vi "Create Response Description.vi"(8 "error in (no error)":errorcluster, 10 "JSON in":string, 11 "Help in":refnum<class "Help.lvclass">) -> (0 "error out":errorcluster, 2 "<JSON> out":string, 3 "Help out":refnum<class "Help.lvclass">)   [LabVIEW 2019, in "Instrument.lvlib" / "Help.lvclass"]
uses:
  Help.lvclass
  Help.lvclass/Help.ctl
  <vilib>/ciozi137/JSON-Schema/API/Read Typedef Description (variant).vi
  <vilib>/JDP Science/JSONtext/JSONtext.lvlib
  <vilib>/ciozi137/JSON-Schema/JSON-Schema.lvlib
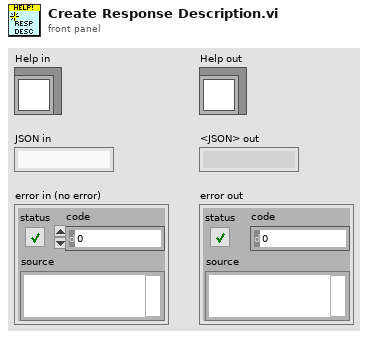
[diagram p1: front panel]
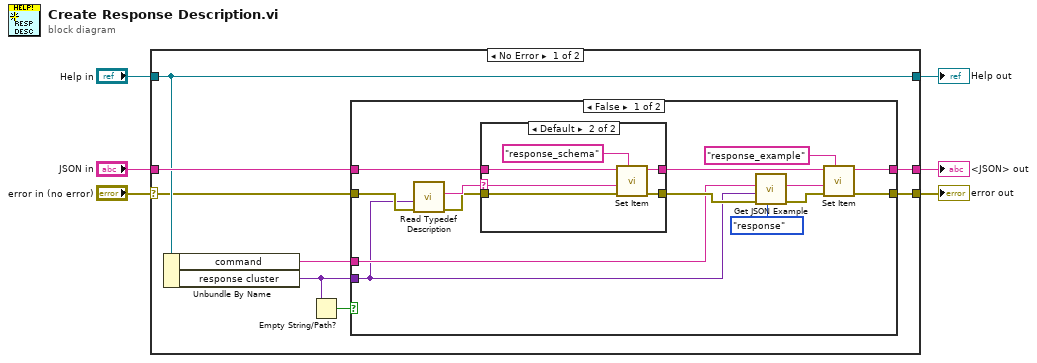
[diagram p0: block diagram]
diagram:
  n1 = case shown="No Error" "error in (no error)" {
    selector: "error in (no error)" -> [w9 w41]
    tunnel: [w14 w39] -> w2
    tunnel: [w13 w41] -> w3
    tunnel: "JSON in" -> [w12 w39]
    tunnel: "Help in" -> [w10 w40]
    tunnel: [w10 w40] -> w6
    frame No Error {
      n2 = Unbundle By Name(w10) -> ("command"=w11:string, "response cluster"=w8:variant)
      n3 = Empty String/Path?(string/path=w8) -> (empty?=w7:bool)
      n4 = case shown="False" w7 {
        tunnel: [w26 w37] -> w14
        tunnel: [w25 w38] -> w13
        tunnel: w12 -> [w24 w37]
        tunnel: w11 -> [w23 _]
        tunnel: w8 -> [w15 _]
        tunnel: w9 -> [w16 w38]
        frame False {
          n5 = call-poly <vilib>:"Read Typedef Description.vi"("error in (no error)"=w16, "variant"=w15) -> ("error out"=w17:errorcluster, "VI description"=w18:string)  [unwired: 7 in, 1 out]
          n6 = case shown="Default" w18 {
            selector: w18 -> [_ w34]
            tunnel: w24 -> [w30 w36]
            tunnel: w17 -> [w29 w35]
            tunnel: [w30 w33] -> w27
            tunnel: [w29 w32] -> w28
            frame "", "{}" {
            }
            frame Default {
              n7 = call <vilib>:"Set Item.vi"("$Path or Item Name"="response_schema", "error in (no error)"=w35, "JSON to Insert"=w34, "JSON"=w36) -> ("error out"=w32:errorcluster, "<JSON>"=w33:string)  [unwired: 4 in, 1 out]
            }
          }
          n8 = call "Get JSON Example.vi"("type"=enum16{"request", "response"}."response", "error in (no error)"=w28, "params or result"=w15, "method"=w23) -> ("error out"=w20:errorcluster, "<JSON>"=w21:string)  [unwired: 6 in]
          n9 = call <vilib>:"Set Item.vi"("$Path or Item Name"="response_example", "error in (no error)"=w20, "JSON to Insert"=w21, "JSON"=w27) -> ("error out"=w25:errorcluster, "<JSON>"=w26:string)  [unwired: 4 in, 1 out]
        }
        frame True {
        }
      }
    }
    frame Error {
    }
  }
  "Help out" <- w6
  "error out" <- w3
  "<JSON> out" <- w2
